vi "Dark Current Right to Folder (SubVI).vi"(6 "Barcodes":string[](array[string]), 9 "Array":dbl[](array[numeric]), 10 "String":string, 11 "appended path":path) -> ()   [LabVIEW 2018]
uses:
  <vilib>/Utility/file.llb/Write Delimited Spreadsheet (string).vi
  <vilib>/Utility/file.llb/Write Delimited Spreadsheet (DBL).vi
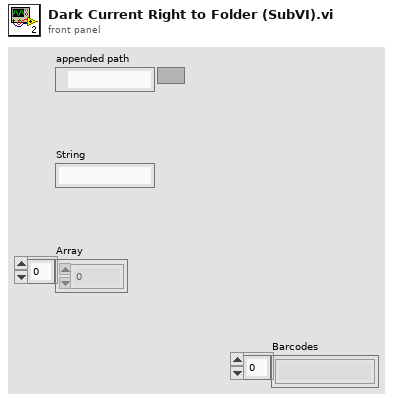
[diagram p1: front panel]
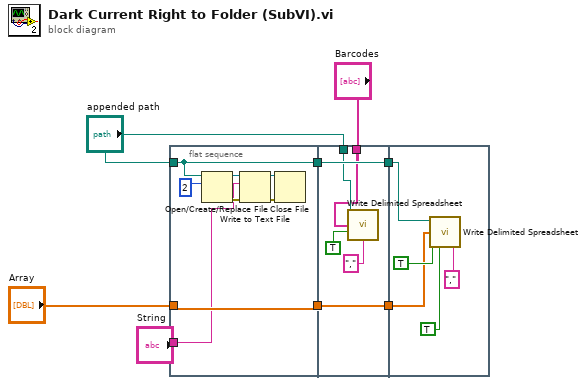
[diagram p0: block diagram]
diagram:
  n1 = flat-sequence {
    tunnel: "appended path" -> [w15]
    tunnel: [w15] -> w8
    tunnel: [w16] -> w7
    tunnel: "Array" -> [w16]
    tunnel: "String" -> [w12]
    tunnel: w8 -> [w22]
    tunnel: [w22] -> w6
    tunnel: w7 -> [w21]
    tunnel: [w21] -> w5
    tunnel: "appended path" -> [w20]
    tunnel: "Barcodes" -> [w19]
    tunnel: w6 -> [w25]
    tunnel: w5 -> [w24]
    frame #0 {
      n2 = Open/Create/Replace File(file path (use dialog)=w15, operation (0:open)=2) -> (refnum out=w13:refnum<file>, error out=w14:errorcluster)  [unwired: 4 in, 1 out]
      n3 = Write to Text File(file (use dialog)=w13, text=w12, error in=w14) -> (refnum out=w10:refnum<file>, error out=w11:errorcluster)  [unwired: 1 in, 1 out]
      n4 = Close File(refnum=w10, error in=w11) -> ()  [unwired: 2 out]
    }
    frame #1 {
      n5 = call-poly <vilib>:"Write Delimited Spreadsheet.vi"("file path (dialog if empty)"=w20, "1D data"=w19, "append to file? (new file:F)"=TRUE, "delimiter (\\t)"=",") -> ()  [unwired: 10 in, 2 out]
    }
    frame #2 {
      n6 = call-poly <vilib>:"Write Delimited Spreadsheet.vi"("file path (dialog if empty)"=w25, "1D data"=w24, "append to file? (new file:F)"=TRUE, "transpose? (no:F)"=TRUE, "delimiter (\\t)"=",") -> ()  [unwired: 9 in, 2 out]
    }
  }
